vi "Configure Session.vi"(8 "error in":errorcluster, 11 "Plugin in":refnum<class "Analog Tachometer Process.lvclass">) -> (0 "error out":errorcluster, 3 "Plugin out":refnum<class "Analog Tachometer Process.lvclass">)   [LabVIEW 2025, in "Analog Tachometer Process.lvlib" / "Analog Tachometer Process.lvclass"]
uses:
  Analog Tachometer Process.lvclass
  C:/Program Files/National Instruments/LabVIEW 2025/vi.lib/FlexLogger/SDK/PluginSDK.lvlibp/PEFClasses/SDK/Plugin/Plugin.lvclass
  Analog Tachometer Process.lvclass/Analog Tachometer Process.ctl
  Helper VIs/Analog Tachometer Process Global.vi
  <vilib>/FlexLogger/SDK/PluginSDK.lvlibp/PEFClasses/SDK/Plugin/ParameterAccess/Read I32.vi
  <vilib>/FlexLogger/SDK/PluginSDK.lvlibp/PEFClasses/SDK/Plugin/ParameterAccess/Write I32.vi
  <vilib>/FlexLogger/SDK/PluginSDK.lvlibp/PEFClasses/SDK/Plugin/ParameterAccess/Read DBL.vi
  <vilib>/FlexLogger/SDK/PluginSDK.lvlibp/PEFClasses/SDK/Plugin/ParameterAccess/Read String.vi
  C:/Program Files/National Instruments/LabVIEW 2025/vi.lib/FlexLogger/SDK/PluginSDK.lvlibp/PEFClasses/SDK/Processing Element/Processing Element.lvclass
  C:/dev/dsb/niflexlogger-plugins/PDK plugins/Analog Tachometer Process/source/Analog Tachometer Process/Analog Tachometer Process.lvclass
  <vilib>/FlexLogger/SDK/PluginSDK.lvlibp/PEFClasses/SDK/Plugin/Plugin.lvclass
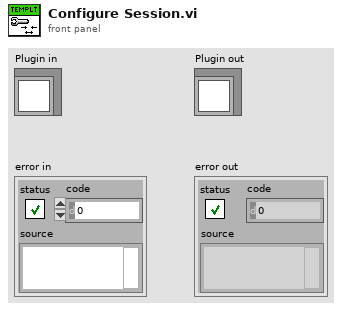
[diagram p1: front panel]
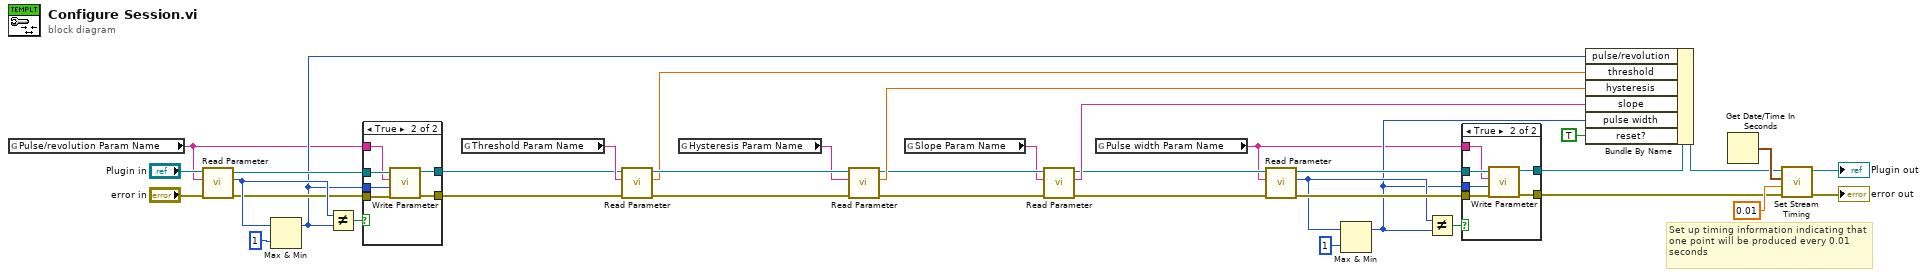
[diagram p0: block diagram]
diagram:
  # "Set up timing information indicating that one point will be produced every 0.01 seconds"
  n1 = global read "Analog Tachometer Process Global.vi" "Pulse/revolution Param Name"() -> (w10:string)
  n2 = call-poly <vilib>:"Read Parameter.vi"("error in (no error)"="error in", "Name"=w10, "Plugin in"="Plugin in") -> ("error out"=w15:errorcluster, "Value"=w16:i32, "Plugin out"=w14:refnum<class "Analog Tachometer Process.lvclass">)  [unwired: 5 in, 1 out]
  n3 = Max & Min(x=w16, y=1) -> (max(x,y)=w11:i32)  [unwired: 1 out]
  n4 = Not Equal?(x=w16, y=w11) -> (x != y?=w17:bool)
  n5 = case shown="True" w17 {
    tunnel: w14 -> [w40 w46]
    tunnel: [w40 w45] -> w13
    tunnel: w15 -> [w39 w44]
    tunnel: w10 -> [_ w43]
    tunnel: w11 -> [_ w42]
    tunnel: [w39 w41] -> w12
    frame False {
    }
    frame True {
      n6 = call-poly <vilib>:"Write Parameter.vi"("error in (no error)"=w44, "Value"=w42, "Name"=w43, "Plugin in"=w46) -> ("error out"=w41:errorcluster, "Plugin out"=w45:refnum<class "Analog Tachometer Process.lvclass">)  [unwired: 6 in]
    }
  }
  n7 = global read "Analog Tachometer Process Global.vi" "Threshold Param Name"() -> (w20:string)
  n8 = call-poly <vilib>:"Read Parameter.vi"("error in (no error)"=w12, "Name"=w20, "Plugin in"=w13) -> ("error out"=w36:errorcluster, "Value"=w32:dbl, "Plugin out"=w34:refnum<class "Analog Tachometer Process.lvclass">)  [unwired: 5 in, 1 out]
  n9 = global read "Analog Tachometer Process Global.vi" "Hysteresis Param Name"() -> (w21:string)
  n10 = call-poly <vilib>:"Read Parameter.vi"("error in (no error)"=w36, "Name"=w21, "Plugin in"=w34) -> ("error out"=w35:errorcluster, "Value"=w33:dbl, "Plugin out"=w30:refnum<class "Analog Tachometer Process.lvclass">)  [unwired: 5 in, 1 out]
  n11 = global read "Analog Tachometer Process Global.vi" "Slope Param Name"() -> (w22:string)
  n12 = call-poly <vilib>:"Read Parameter.vi"("error in (no error)"=w35, "Name"=w22, "Plugin in"=w30) -> ("error out"=w31:errorcluster, "Value"=w29:string, "Plugin out"=w28:refnum<class "Analog Tachometer Process.lvclass">)  [unwired: 5 in, 1 out]
  n13 = global read "Analog Tachometer Process Global.vi" "Pulse width Param Name"() -> (w3:string)
  n14 = call-poly <vilib>:"Read Parameter.vi"("error in (no error)"=w31, "Name"=w3, "Plugin in"=w28) -> ("error out"=w8:errorcluster, "Value"=w5:i32, "Plugin out"=w6:refnum<class "Analog Tachometer Process.lvclass">)  [unwired: 5 in, 1 out]
  n15 = Max & Min(x=w5, y=1) -> (max(x,y)=w4:i32)  [unwired: 1 out]
  n16 = Not Equal?(x=w5, y=w4) -> (x != y?=w9:bool)
  n17 = case shown="True" w9 {
    tunnel: w6 -> [w48 w54]
    tunnel: [w48 w53] -> w7
    tunnel: w8 -> [w47 w52]
    tunnel: w3 -> [_ w51]
    tunnel: w4 -> [_ w50]
    tunnel: [w47 w49] -> w2
    frame False {
    }
    frame True {
      n18 = call-poly <vilib>:"Write Parameter.vi"("error in (no error)"=w52, "Value"=w50, "Name"=w51, "Plugin in"=w54) -> ("error out"=w49:errorcluster, "Plugin out"=w53:refnum<class "Analog Tachometer Process.lvclass">)  [unwired: 6 in]
    }
  }
  n19 = Bundle By Name(cluster=w7, "pulse/revolution"=w11, "threshold"=w32, "hysteresis"=w33, "slope"=w29, "pulse width"=w4, "reset?"=TRUE) -> (w1:refnum<class "Analog Tachometer Process.lvclass">)
  n20 = Get Date/Time In Seconds() -> (seconds since 1Jan1904=w26:timestamp)
  n21 = call-dynamic "Set Stream Timing.vi"("error in (no error)"=w2, "dt(sec)"=0.01, "Start Time"=w26, "Plugin in"=w1) -> ("error out"=→"error out":errorcluster, "Plugin out"=→"Plugin out":refnum<class "Analog Tachometer Process.lvclass">)  [unwired: 6 in]
